vi "linfit.vi"() -> ()   [LabVIEW 2019]
uses:
  <vilib>/Analysis/NI_AALPro.lvlib
panel:
  out "XY Graph":cluster{"U":dbl[], "P":dbl[]}[](graph)=[{"U"=[0.4, 0.5, 0.6, 0.7, 0.75, 0.8], "P"=[18.39, 24.68, 31.59, 38.46, 42.35, 45.56]}, {"U"=[0.4, 0.5, 0.6, 0.7, 0.75, 0.8], "P"=[18.39, 24.68, 31.59, 38.46, 42.35, 45.56]}]
  out "residue 2":dbl=0.28076937818829606
  out "intercept 2":dbl=-6.637213566799896
  out "slope 2":dbl=67.84599476078859
  out "residue":dbl=0.052654385964880625
  out "intercept":dbl=-9.33052631578932
  out "slope":dbl=68.53684210526293
  in  "Pair":dbl[](array[numeric])=[0.36, 0.47, 0.57, 0.67, 0.71, 0.77]
  in  "U":dbl[](array[numeric])=[0.4, 0.5, 0.6, 0.7, 0.75, 0.8]
  in  "P":dbl[](array[numeric])=[18.39, 24.68, 31.59, 38.46, 42.35, 45.56]
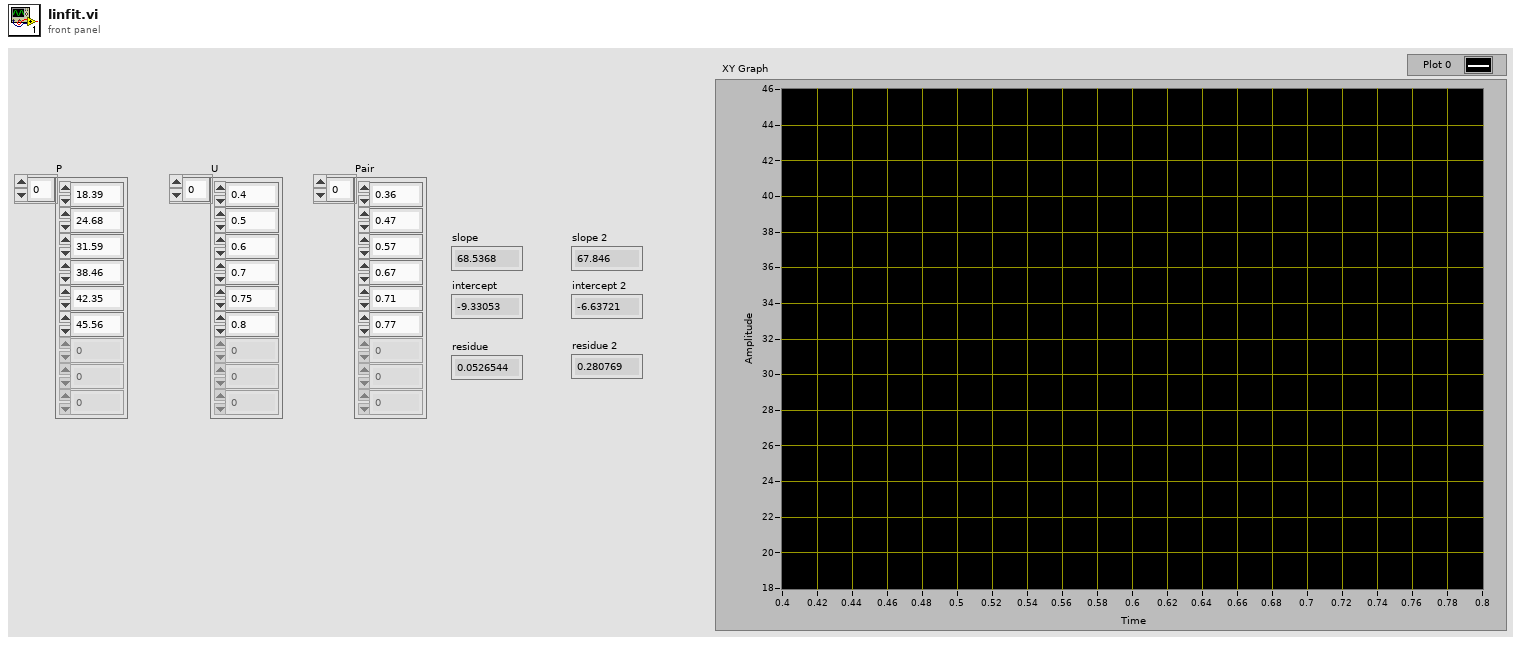
[diagram p1: front panel]
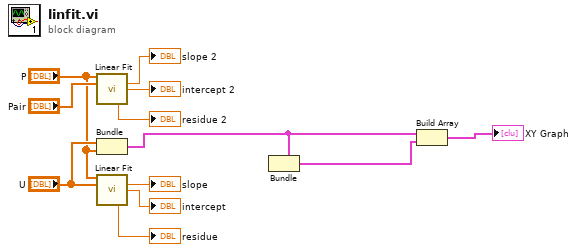
[diagram p0: block diagram]
diagram:
  n1 = call <vilib>:"Linear Fit.vi"("Y"="P", "X"="Pair") -> ("slope"=→"slope 2":dbl, "intercept"=→"intercept 2":dbl, "residue"=→"residue 2":dbl)  [unwired: 9 in, 2 out]
  n2 = Bundle("U"="U", "P"="P") -> (w3:cluster{"U":dbl[], "P":dbl[]})  [unwired: 1 in]
  n3 = call <vilib>:"Linear Fit.vi"("Y"="P", "X"="U") -> ("slope"=→"slope":dbl, "intercept"=→"intercept":dbl, "residue"=→"residue":dbl)  [unwired: 9 in, 2 out]
  n4 = Bundle(cluster=w3) -> (w1:cluster{"U":dbl[], "P":dbl[]})  [unwired: 2 in]
  n5 = Build Array(w3, w1) -> (→"XY Graph":cluster{"U":dbl[], "P":dbl[]}[])
